vi "SingleCounter-trig_start_stop.vi"(10 "Duration_s":dbl=0.0003) -> (0 "error out":errorcluster, 1 "triggers_task":refnum<k21>, 2 "Waveform Graph":u32[](graph), 3 "APD_task":refnum<k21>)   [LabVIEW 2018]
uses:
  GLOBAL_VAR.vi
  <vilib>/DAQmx/create/channels.llb/DAQmx Create Channel (CI-Count Edges).vi
  <vilib>/DAQmx/configure/timing.llb/DAQmx Timing (Sample Clock).vi
  <resource>/objmgr/daqmx.rc
  <vilib>/DAQmx/read.llb/DAQmx Read (Counter 1D U32 1Chan NSamp).vi
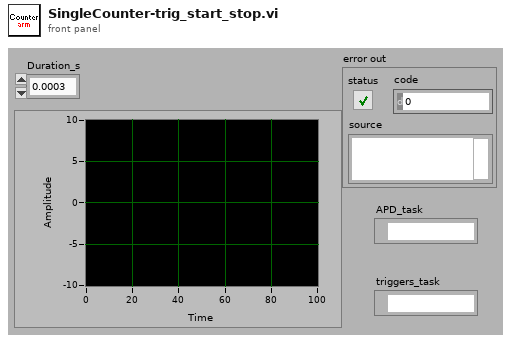
[diagram p1: front panel]
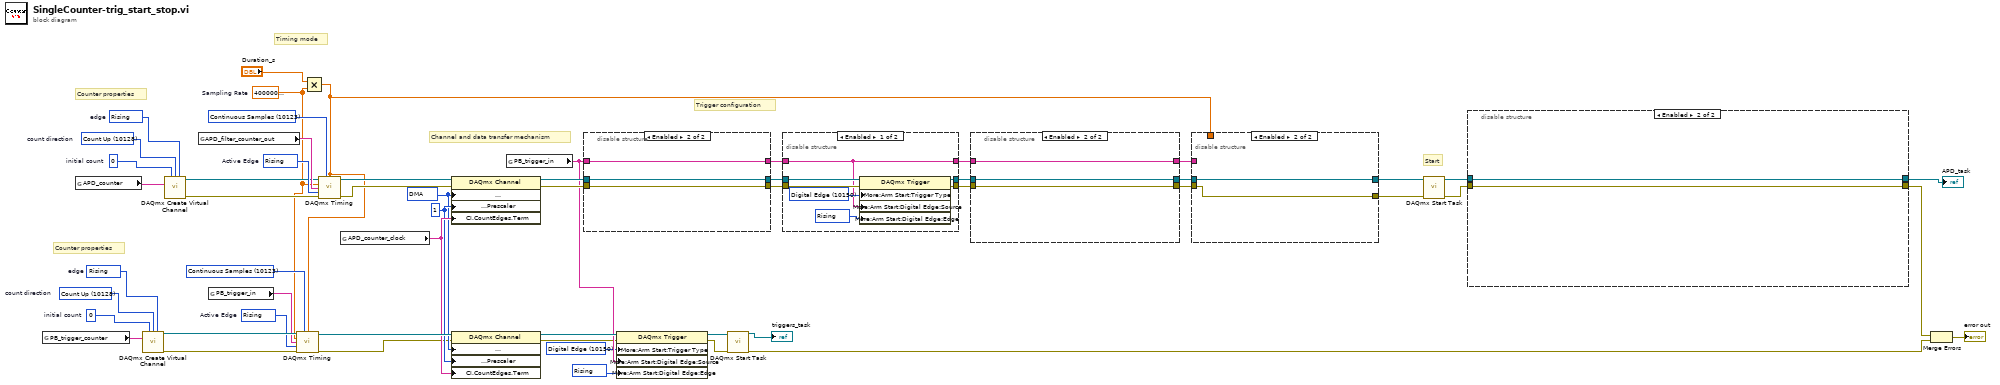
[diagram p0: block diagram]
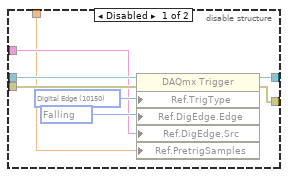
[diagram p2: hidden frame]
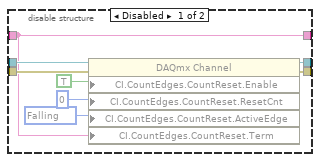
[diagram p4: hidden frame]
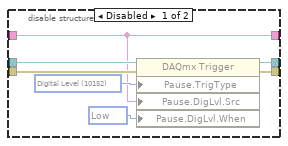
[diagram p5: hidden frame]
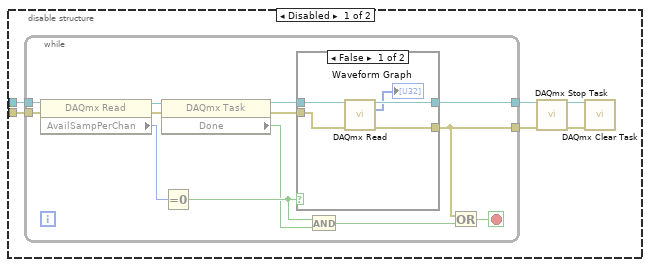
[diagram p6: hidden frame]
diagram:
  w10 = 10150 items=["Digital Edge"=10150, "None"=10230] ("Trigger Type")
  w9 = 10280 items=["Rising"=10280, "Falling"=10171] ("Trigger Edge")
  w22 = 10280 items=["Rising"=10280, "Falling"=10171]  # Active Edge
  w20 = 10123 items=["Finite Samples"=10178, "Continuous Samples"=10123, "Hardware Timed Single Point"=12522] ("Sample Mode")
  w26 = 10128 items=["Count Up"=10128, "Count Down"=10124, "Externally Controlled"=10326]  # count direction
  w27 = 10280 items=["Rising"=10280, "Falling"=10171]  # edge
  w25 = u32 0  # initial count
  w19 = 40000000.0  # Sampling Rate
  w14 = u32 1 ("CI.Prescaler")
  w55 = 10280 items=["Rising"=10280, "Falling"=10171]  # Active Edge
  w53 = 10128 items=["Count Up"=10128, "Count Down"=10124, "Externally Controlled"=10326]  # count direction
  w54 = 10280 items=["Rising"=10280, "Falling"=10171]  # edge
  w52 = u32 0  # initial count
  w13 = 10054 items=["DMA"=10054, "Interrupts"=10204, "Programmed I/O"=10264] ("CI.DataXferMech")
  w51 = 10123 items=["Finite Samples"=10178, "Continuous Samples"=10123, "Hardware Timed Single Point"=12522] ("Sample Mode")
  # "Counter properties"
  # "Trigger configuration"
  # "Counter properties"
  # "Channel and data transfer mechanism"
  # "Timing mode"
  # "Start"
  n1 = global read "GLOBAL_VAR.vi" "PB_trigger_counter"() -> (w24:tag)
  n2 = global read "GLOBAL_VAR.vi" "APD_counter"() -> (w47:tag)
  n3 = call-poly <vilib>:"DAQmx Create Virtual Channel.vi"("initial count"=w25, "count direction"=w26, "edge"=w27, "counter"=w24) -> ("task out"=w23:refnum<k21>, "error out"=w17:errorcluster)  [unwired: 10 in]
  n4 = call-poly <vilib>:"DAQmx Create Virtual Channel.vi"("initial count"=w52, "count direction"=w53, "edge"=w54, "counter"=w47) -> ("task out"=w45:refnum<k21>, "error out"=w44:errorcluster)  [unwired: 10 in]
  n5 = global read "GLOBAL_VAR.vi" "APD_filter_counter_out"() -> (w46:tag)
  n6 = global read "GLOBAL_VAR.vi" "PB_trigger_in"() -> (w21:tag)
  n7 = Multiply(x="Duration_s", y=w19) -> (x*y=w18:dbl)
  n8 = call-poly <vilib>:"DAQmx Timing.vi"("task/channels in"=w23, "sample mode"=w20, "samples per channel"=w18, "rate"=w19, "source"=w21, "active edge"=w22, "error in"=w17) -> ("task out"=w16:refnum<k21>, "error out"=w5:errorcluster)  [unwired: 7 in]
  n9 = call-poly <vilib>:"DAQmx Timing.vi"("task/channels in"=w45, "sample mode"=w51, "samples per channel"=w18, "rate"=w19, "source"=w46, "active edge"=w55, "error in"=w44) -> ("task out"=w42:refnum<k21>, "error out"=w43:errorcluster)  [unwired: 7 in]
  n10 = global read "GLOBAL_VAR.vi" "APD_counter_clock"() -> (w15:tag)
  n11 = property class="DAQmx Channel"(reference=w42, error in=w43, "Counter Input:General Properties:More:Advanced:Data Transfer and Memory:Data Transfer Mechanism"=w13, "Counter Input:General Properties:More:Advanced:Prescaler"=w14, "CI.CountEdges.Term"=w15) -> (reference out=w38:refnum<k21>, error out=w37:errorcluster)
  n12 = property class="DAQmx Channel"(reference=w16, error in=w5, "Counter Input:General Properties:More:Advanced:Data Transfer and Memory:Data Transfer Mechanism"=w13, "Counter Input:General Properties:More:Advanced:Prescaler"=w14, "CI.CountEdges.Term"=w15) -> (reference out=w12:refnum<k21>, error out=w6:errorcluster)
  n13 = global read "GLOBAL_VAR.vi" "PB_trigger_in"() -> (w11:tag)
  n14 = disable-structure shown="Enabled" {
    disable-tunnel: w38 -> [w62 w65]
    disable-tunnel: w37 -> [w61 w64]
    disable-tunnel: [w58 w65] -> w36
    disable-tunnel: [w57 w64] -> w35
    disable-tunnel: [w56 w63] -> w28
    disable-tunnel: w11 -> [w56 w63]
    frame Disabled {
      w59 = 10214 items=["High"=10192, "Low"=10214] ("Pause.DigLvl.When")
      w60 = 10152 items=["Analog Level"=10101, "Analog Window"=10103, "Digital Level"=10152, "Digital Pattern"=10398, "None"=10230] ("Pause.TrigType")
      n15 = property class="DAQmx Trigger"(reference=w62, error in=w61, "Pause.TrigType"=w60, "Pause.DigLvl.Src"=w56, "Pause.DigLvl.When"=w59) -> (reference out=w58:refnum<k21>, error out=w57:errorcluster)
    }
    frame Enabled {
    }
  }
  n16 = property class="DAQmx Trigger"(reference=w12, error in=w6, "More:Arm Start:Trigger Type"=w10, "More:Arm Start:Digital Edge:Source"=w11, "More:Arm Start:Digital Edge:Edge"=w9) -> (reference out=w8:refnum<k21>, error out=w7:errorcluster)
  n17 = call <vilib>:"DAQmx Start Task.vi"("task/channels in"=w8, "error in"=w7) -> ("task out"=→"triggers_task":refnum<k21>, "error out"=w1:errorcluster)  [unwired: 12 in]
  n18 = disable-structure shown="Enabled" {
    disable-tunnel: [w72 w75] -> w40
    disable-tunnel: [w71 w74] -> w39
    disable-tunnel: w36 -> [w70 w75]
    disable-tunnel: w35 -> [w69 w74]
    disable-tunnel: w28 -> [w66 w73]
    disable-tunnel: [w66 w73] -> w29
    frame Enabled {
      w68 = 10150 items=["Digital Edge"=10150, "None"=10230] ("Trigger Type")
      w67 = 10280 items=["Rising"=10280, "Falling"=10171] ("Trigger Edge")
      n19 = property class="DAQmx Trigger"(reference=w70, error in=w69, "More:Arm Start:Trigger Type"=w68, "More:Arm Start:Digital Edge:Source"=w66, "More:Arm Start:Digital Edge:Edge"=w67) -> (reference out=w72:refnum<k21>, error out=w71:errorcluster)
    }
    frame Disabled {
    }
  }
  n20 = disable-structure shown="Enabled" {
    disable-tunnel: w40 -> [w83 w86]
    disable-tunnel: w39 -> [w82 w85]
    disable-tunnel: [w81 w86] -> w34
    disable-tunnel: [w80 w85] -> w33
    disable-tunnel: w29 -> [w76 w84]
    disable-tunnel: [w76 w84] -> w30
    frame Disabled {
      w77 = 10171 items=["Rising"=10280, "Falling"=10171] ("CI.CountEdges.CountReset.ActiveEdge")
      n21 = property class="DAQmx Channel"(reference=w83, error in=w82, "CI.CountEdges.CountReset.Enable"=TRUE, "CI.CountEdges.CountReset.ResetCnt"=u32 0, "CI.CountEdges.CountReset.ActiveEdge"=w77, "CI.CountEdges.CountReset.Term"=w76) -> (reference out=w81:refnum<k21>, error out=w80:errorcluster)
    }
    frame Enabled {
    }
  }
  n22 = disable-structure shown="Enabled" {
    disable-tunnel: w34 -> [w94 w96]
    disable-tunnel: w33 -> [w93 w95]
    disable-tunnel: [w90 w96] -> w32
    disable-tunnel: [w87 w95] -> w31
    disable-tunnel: w30 -> [w89 _]
    disable-tunnel: w18 -> [w88 _]
    frame Disabled {
      w91 = 10171 items=["Rising"=10280, "Falling"=10171] ("Ref.DigEdge.Edge")
      w92 = 10150 items=["Analog Edge"=10099, "Digital Edge"=10150, "Digital Pattern"=10398, "Analog Window"=10103, "None"=10230] ("Ref.TrigType")
      n23 = property class="DAQmx Trigger"(reference=w94, error in=w93, "Ref.TrigType"=w92, "Ref.DigEdge.Edge"=w91, "Ref.DigEdge.Src"=w89, "Ref.PretrigSamples"=w88) -> (reference out=w90:refnum<k21>, error out=w87:errorcluster)
    }
    frame Enabled {
    }
  }
  n24 = call <vilib>:"DAQmx Start Task.vi"("task/channels in"=w32, "error in"=w31) -> ("task out"=w48:refnum<k21>, "error out"=w49:errorcluster)  [unwired: 12 in]
  n25 = disable-structure shown="Enabled" {
    disable-tunnel: w49 -> [w102 w123]
    disable-tunnel: w48 -> [w101 w124]
    disable-tunnel: [_ w124] -> w41
    disable-tunnel: [_ w123] -> w3
    frame Disabled {
      n26 = while {
        tunnel: w102 -> [w113]
        tunnel: w101 -> [w112]
        tunnel: [w108] -> w98
        tunnel: [w106] -> w97
        stop <- w107 stop-if-true
        n27 = property class="DAQmx Read"(reference=w112, error in=w113) -> (reference out=w115:refnum<k21>, error out=w114:errorcluster, "AvailSampPerChan"=w111:u32)
        n28 = property class="DAQmx Task"(reference=w115, error in=w114) -> (reference out=w110:refnum<k21>, error out=w109:errorcluster, "Done"=w103:bool)
        n29 = Equal To 0?(x=w111) -> (x = 0?=w104:bool)
        n30 = case shown="False" w104 {
          tunnel: w110 -> [w120 w122]
          tunnel: w109 -> [w119 w121]
          tunnel: [w118 w122] -> w108
          tunnel: [w117 w121] -> w106
          frame False {
            n31 = call-poly <vilib>:"DAQmx Read.vi"("task/channels in"=w120, "error in"=w119) -> ("task out"=w118:refnum<k21>, "data"=→"Waveform Graph":u32[], "error out"=w117:errorcluster)  [unwired: 11 in]
          }
          frame True {
          }
        }
        n32 = And(x=w104, y=w103) -> (x .and. y?=w105:bool)
        n33 = Or(x=w106, y=w105) -> (x .or. y?=w107:bool)
      }
      n34 = call <vilib>:"DAQmx Stop Task.vi"("task/channels in"=w98, "error in"=w97) -> ("task out"=w100:refnum<k21>, "error out"=w99:errorcluster)  [unwired: 12 in]
      n35 = call <vilib>:"DAQmx Clear Task.vi"("task in"=w100, "error in"=w99) -> ()  [unwired: 13 in, 1 out]
    }
    frame Enabled {
    }
  }
  "APD_task" <- w41
  n36 = Merge Errors(w3, w1) -> (→"error out":errorcluster)
